vi "Override Error.vi"(10 "Error":errorcluster, 11 "Base Event jettl in":refnum<class "Base Event jettl.lvclass">) -> (3 "Base Event jettl out":refnum<class "Base Event jettl.lvclass">)   [LabVIEW 2021, in "jettl.lvlib" / "Base Event jettl.lvlib" / "Base Event jettl.lvclass"]
uses:
  Base Event jettl.lvclass
  Base Event jettl.lvclass/Base Event jettl.ctl
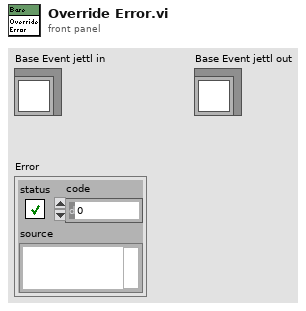
[diagram p1: front panel]
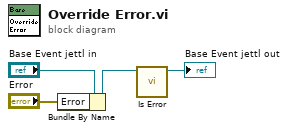
[diagram p0: block diagram]
diagram:
  n1 = Bundle By Name(cluster="Base Event jettl in", "Error"="Error") -> (w2:refnum<class "Base Event jettl.lvclass">)
  n2 = call "Is Error.vi"("Base Event jettl in"=w2) -> ("Base Event jettl out"=→"Base Event jettl out":refnum<class "Base Event jettl.lvclass">)  [unwired: 10 in]
